vi "Test Lockin Proc.vi"() -> ()   [LabVIEW 2021]
uses:
  NHMFL_Core/Libraries/SoftwareLockin/Lockin Parameters.ctl
  NHMFL_Core/Libraries/SoftwareLockin/Lock-in Detector/Lock-in Detector.lvclass
  NHMFL_Core/Libraries/SoftwareLockin/Software Lock-in/Software Lock-in.lvclass
  NHMFL_Core/Libraries/SoftwareLockin/Lock-in Detector/Lock-in Detector.lvclass/Lock-in Detector.ctl
  NHMFL_Core/Libraries/SoftwareLockin/Lock-in Detector/Write Reference amplitude.vi
  NHMFL_Core/Libraries/SoftwareLockin/Lock-in Detector/Write Reference frequency.vi
  NHMFL_Core/Libraries/SoftwareLockin/Lock-in Detector/Write Sample rate.vi
  NHMFL_Core/Libraries/SoftwareLockin/Lock-in Detector/Write Time constant.vi
  <vilib>/Analysis/NI_AALBase.lvlib
panel:
  in  "Width":dbl=1.0
  out "Waveform Graph 3":dbl[](graph)
  out "Waveform Graph 2":dbl[](graph)
  in  "Time constant":dbl=0.0001 format="%#_6ps"
  out "Waveform Graph":dbl[](graph)
  in  "Sample rate":dbl=3333333.33 format="%#_6pHz"
  in  "Duration":dbl=0.09999999999999998 format="%#_6ps"
  in  "Lockin parameters":T1={"Frequency"=127000.0, "Phase"=0.0, "Syncronous"=FALSE, "Points per sine wave"=0, "DDS"=FALSE, "Frequency word"=0, "Phase word"=0, "DDS modulus"=15120, "DDS clock"=125000000.0} {"DDS clock" format="%_17pHz"; "DDS modulus" format="0x%x (%d)"; "Phase" format="%#_gdeg"; "Frequency" format="%_17pHz"}
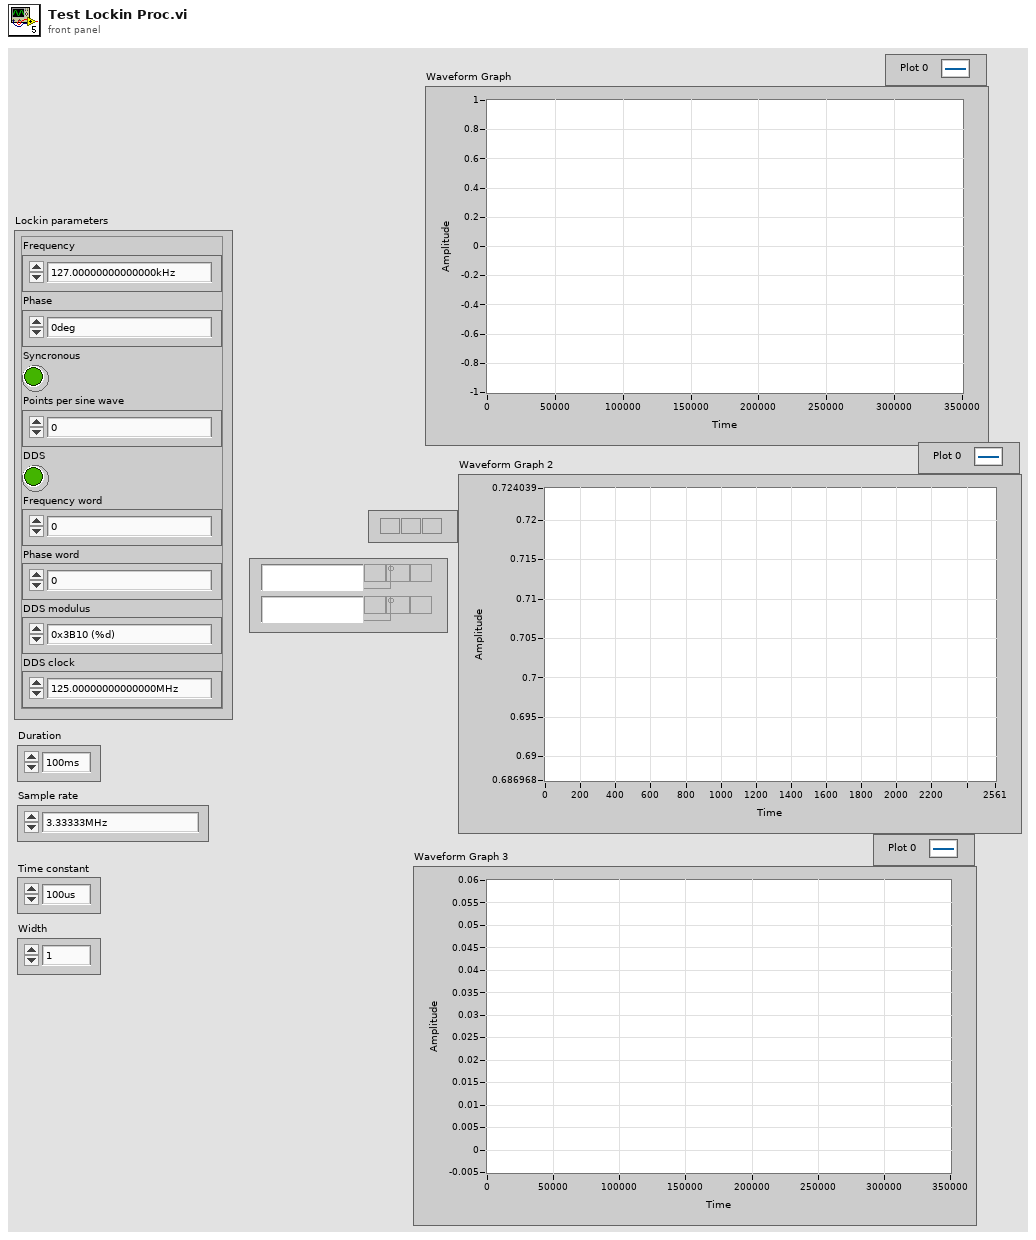
[diagram p1: front panel]
types:
  T1 = typedef "Lockin Parameters.ctl" = cluster{"Frequency":dbl, "Phase":dbl, "Syncronous":bool, "Points per sine wave":i32, "DDS":bool, "Frequency word":u32, "Phase word":u32, "DDS modulus":i64, "DDS clock":dbl}
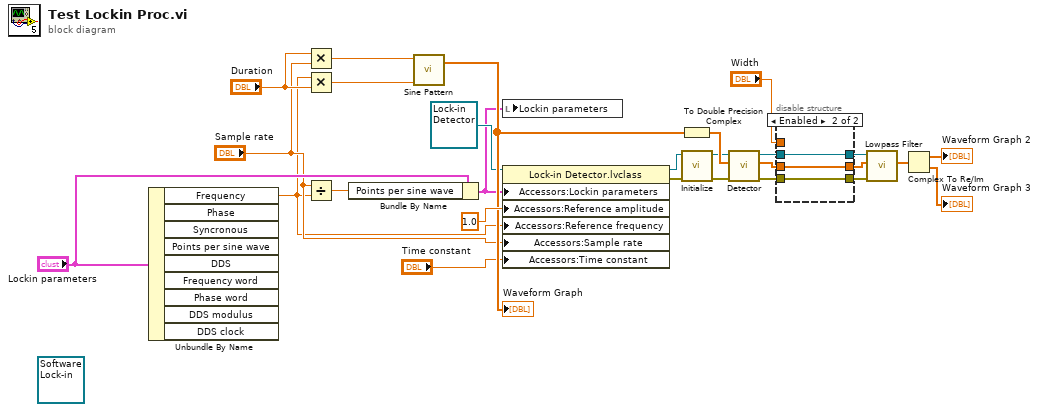
[diagram p0: block diagram]
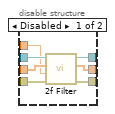
[diagram p2: hidden frame]
diagram:
  (unwired) refnum<class "Software Lock-in.lvclass"> refnum ("Software Lock-in in")
  n1 = Unbundle By Name("Lockin parameters") -> ("Frequency"=w13:dbl)  [unwired: 8 out]
  n2 = Multiply(x="Duration", y="Sample rate") -> (x*y=w27:dbl)
  n3 = Multiply(x=w13, y="Duration") -> (x*y=w25:dbl)
  n4 = Divide(x="Sample rate", y=w13) -> (x/y=w12:dbl)
  n5 = Bundle By Name(cluster="Lockin parameters", "Points per sine wave"=w12) -> (w11:T1)
  n6 = call <vilib>:"Sine Pattern.vi"("cycles"=w25, "samples"=w27) -> ("Sinusoidal Pattern"=w23:dbl[])  [unwired: 2 in, 1 out]
  "Waveform Graph" <- w23
  n7 = local write "Lockin parameters"(w11) -> ()
  n8 = property class="Lock-in Detector.lvclass"(reference=refnum<class "Lock-in Detector.lvclass"> refnum ("Lock-in Detector in"), "Accessors:Lockin parameters"=w11, "Accessors:Reference amplitude"=1.0 ("Reference amplitude"), "Accessors:Reference frequency"=w13, "Accessors:Sample rate"="Sample rate", "Accessors:Time constant"="Time constant") -> (reference out=w20:refnum<class "Lock-in Detector.lvclass">, error out=w18:errorcluster)  [unwired: 1 in]
  n9 = To Double Precision Complex(1:w23) -> (0:w22:cdb[])
  n10 = call-dynamic "Initialize.vi"("error in (no error)"=w18, "Software Lock-in in"=w20) -> ("error out"=w16:errorcluster, "Software Lock-in out"=w17:refnum<class "Lock-in Detector.lvclass">)  [unwired: 7 in, 1 out]
  n11 = call-dynamic "Detector.vi"("error in (no error)"=w16, "Signal"=w22, "Lock-in Detector in"=w17) -> ("error out"=w7:errorcluster, "Signal out"=w3:cdb[], "Lock-in Detector out"=w5:refnum<class "Lock-in Detector.lvclass">)  [unwired: 6 in]
  n12 = disable-structure shown="Enabled" {
    disable-tunnel: w7 -> [w34 w36]
    disable-tunnel: [w33 w36] -> w6
    disable-tunnel: w5 -> [w32 w37]
    disable-tunnel: [w31 w37] -> w4
    disable-tunnel: w3 -> [w30 w35]
    disable-tunnel: [w29 w35] -> w2
    disable-tunnel: "Width" -> [w28 _]
    frame Disabled {
      n13 = call-dynamic "2f Filter.vi"("error in (no error)"=w34, "Width"=w28, "Signal"=w30, "Lock-in Detector in"=w32) -> ("error out"=w33:errorcluster, "Signal out"=w29:cdb[], "Lock-in Detector out"=w31:refnum<class "Lock-in Detector.lvclass">)  [unwired: 5 in]
    }
    frame Enabled {
    }
  }
  n14 = call-dynamic "Lowpass Filter.vi"("error in (no error)"=w6, "Signal"=w2, "Lock-in Detector in"=w4) -> ("Signal out"=w8:cdb[])  [unwired: 6 in, 2 out]
  n15 = Complex To Re/Im(x + iy=w8) -> (x=→"Waveform Graph 2":dbl[], y=→"Waveform Graph 3":dbl[])
